vi "IO_MFA_DOUT_Read_DigitalOutput1.vi"(9 "O/P Actlevel1":bool, 11 "O/P Actlevel0":bool) -> (0 "OutputActiveLevel 1":i32, 1 "ErrorActLvl1":bool, 2 "OutputActiveLevel 0":i32, 3 "ErrorActLvl0":bool)   [LabVIEW 2018]
panel:
  out "error DriveOuput Check Off":errorcluster
  out "error DriveOuput Check On":errorcluster
  out "error DriveOutput Off":errorcluster
  out "error DriveOutput On":errorcluster
  out "AAABuild":i32
  in  "MintController":refnum<k7>(container)
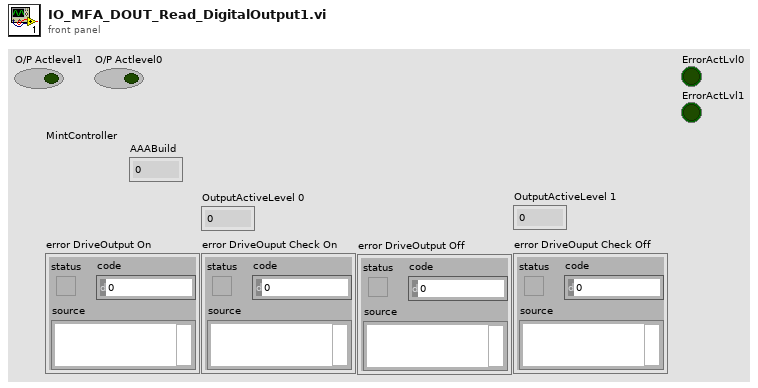
[diagram p1: front panel]
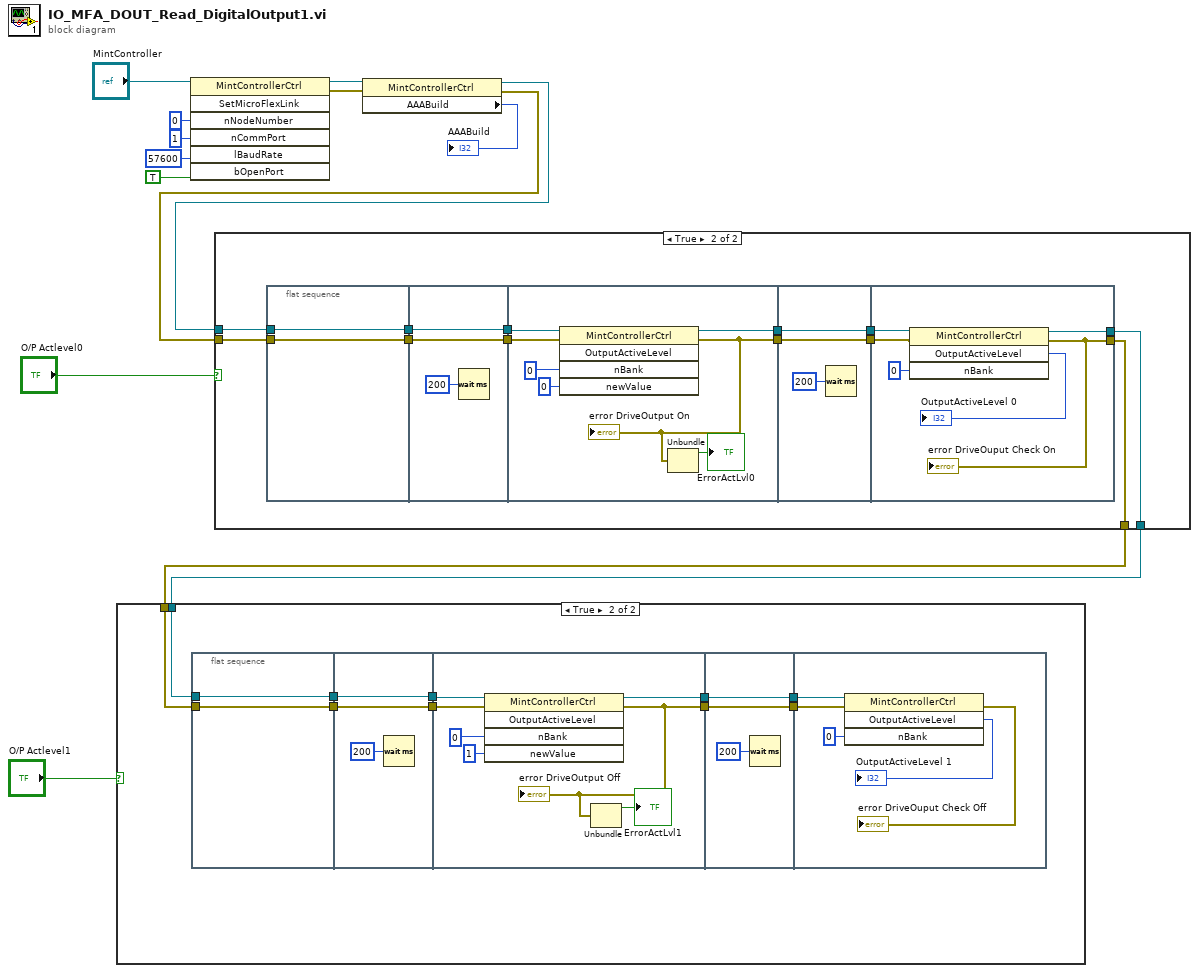
[diagram p0: block diagram]
diagram:
  n1 = invoke class="MintControllerCtrl" method="SetMicroFlexLink"(reference="MintController", "nNodeNumber"=i16 0, "nCommPort"=i16 1, "lBaudRate"=57600, "bOpenPort"=TRUE) -> (reference out=w14:refnum<k7>, error out=w8:errorcluster)  [unwired: 2 in, 5 out]
  n2 = property class="MintControllerCtrl"(reference=w14, error in=w8) -> (reference out=w5:refnum<k7>, error out=w6:errorcluster, "AAABuild"=→"AAABuild":i32)
  n3 = case shown="True" "O/P Actlevel0" {
    tunnel: w6 -> [w15 w20]
    tunnel: w5 -> [w16 w19]
    tunnel: [w16 w18] -> w4
    tunnel: [w15 w17] -> w3
    frame False {
    }
    frame True {
      n4 = flat-sequence {
        tunnel: w19 -> [w29]
        tunnel: w20 -> [w30]
        tunnel: [w30] -> w28
        tunnel: [w29] -> w27
        tunnel: [w33] -> w26
        tunnel: [w32] -> w25
        tunnel: w28 -> [w33]
        tunnel: w27 -> [w32]
        tunnel: w26 -> [w39]
        tunnel: w25 -> [w38]
        tunnel: [w36] -> w24
        tunnel: [w35] -> w23
        tunnel: w24 -> [w43]
        tunnel: w23 -> [w42]
        tunnel: [w43] -> w22
        tunnel: [w42] -> w21
        tunnel: w22 -> [w49]
        tunnel: w21 -> [w48]
        tunnel: [w45] -> w18
        tunnel: [w44] -> w17
        frame #0 {
        }
        frame #1 {
          n5 = Wait (ms)(milliseconds to wait=u32 200) -> ()  [unwired: 1 out]
        }
        frame #2 {
          n6 = invoke class="MintControllerCtrl" method="OutputActiveLevel"(reference=w38, error in=w39, "nBank"=i16 0 ("nAxis"), "newValue"=0) -> (reference out=w36:refnum<k7>, error out=w35:errorcluster)  [unwired: 1 in, 3 out]
          "error DriveOutput On" <- w35
          n7 = Unbundle(w35) -> ("status"=→"ErrorActLvl0":bool)  [unwired: 2 out]
        }
        frame #3 {
          n8 = Wait (ms)(milliseconds to wait=u32 200) -> ()  [unwired: 1 out]
        }
        frame #4 {
          n9 = invoke class="MintControllerCtrl" method="OutputActiveLevel"(reference=w49, error in=w48, "nBank"=i16 0) -> (reference out=w45:refnum<k7>, error out=w44:errorcluster, "OutputActiveLevel"=→"OutputActiveLevel 0":i32)  [unwired: 1 in, 1 out]
          "error DriveOuput Check On" <- w44
        }
      }
    }
  }
  n10 = case shown="True" "O/P Actlevel1" {
    tunnel: w4 -> [_ w51]
    tunnel: w3 -> [_ w50]
    frame False {
    }
    frame True {
      n11 = flat-sequence {
        tunnel: w51 -> [w60]
        tunnel: w50 -> [w61]
        tunnel: [w61] -> w59
        tunnel: [w60] -> w58
        tunnel: [w64] -> w57
        tunnel: [w63] -> w56
        tunnel: w59 -> [w64]
        tunnel: w58 -> [w63]
        tunnel: w57 -> [w70]
        tunnel: w56 -> [w69]
        tunnel: [w66] -> w55
        tunnel: [w67] -> w54
        tunnel: [w73] -> w53
        tunnel: w55 -> [w73]
        tunnel: [w72] -> w52
        tunnel: w54 -> [w72]
        tunnel: w53 -> [w79]
        tunnel: w52 -> [w78]
        frame #0 {
        }
        frame #1 {
          n12 = Wait (ms)(milliseconds to wait=u32 200) -> ()  [unwired: 1 out]
        }
        frame #2 {
          n13 = invoke class="MintControllerCtrl" method="OutputActiveLevel"(reference=w69, error in=w70, "nBank"=i16 0 ("nAxis"), "newValue"=1) -> (reference out=w67:refnum<k7>, error out=w66:errorcluster)  [unwired: 1 in, 3 out]
          "error DriveOutput Off" <- w66
          n14 = Unbundle(w66) -> ("status"=→"ErrorActLvl1":bool)  [unwired: 2 out]
        }
        frame #3 {
          n15 = Wait (ms)(milliseconds to wait=u32 200) -> ()  [unwired: 1 out]
        }
        frame #4 {
          n16 = invoke class="MintControllerCtrl" method="OutputActiveLevel"(reference=w78, error in=w79, "nBank"=i16 0) -> (error out=→"error DriveOuput Check Off":errorcluster, "OutputActiveLevel"=→"OutputActiveLevel 1":i32)  [unwired: 1 in, 2 out]
        }
      }
    }
  }
